vi "AndorSet.vi"(8 "error in":errorcluster, 9 "MultiTrack":cluster{"StartRow":i32, "EndRow":i32}={"StartRow"=1, "EndRow"=256}, 10 "AcqSet":T2={"openingtime"=20, "closingtime"=20, "ExposureTime"=0.01, "AccumCycTime"=0.0, "AccumCycNum"=1, "KineticNum"=1, "KineticTime"=0.0} {"KineticTime" format="%.2f"; "AccumCycTime" format="%.2f"; "ExposureTime" format="%.2f"}, 11 "Mode":T8={"AcqMode"=enum."Single Scan", "ReadMode"=enum."Image", "ShutterMode"=enum."Auto", "GateMode"=enum."TTL High", "TriggerMode"=enum."Internal"}) -> (0 "error out":errorcluster, 1 "SetStatus":bool, 2 "SetOut":T9, 3 "Timing":T1 {"kinetic" format="%.2f"; "accumulate" format="%.2f"; "exposure" format="%.2f"})   [LabVIEW 2014]
uses:
  <userlib>/atmcd64d.llb/AcquisitionMode_mode typedef.ctl
  <userlib>/atmcd64d.llb/ReadMode_mode typedef.ctl
  <userlib>/atmcd64d.llb/Shutter_mode typedef.ctl
  <userlib>/atmcd64d.llb/Shutter_type typedef.ctl
  <userlib>/atmcd64d.llb/TriggerMode_mode typedef.ctl
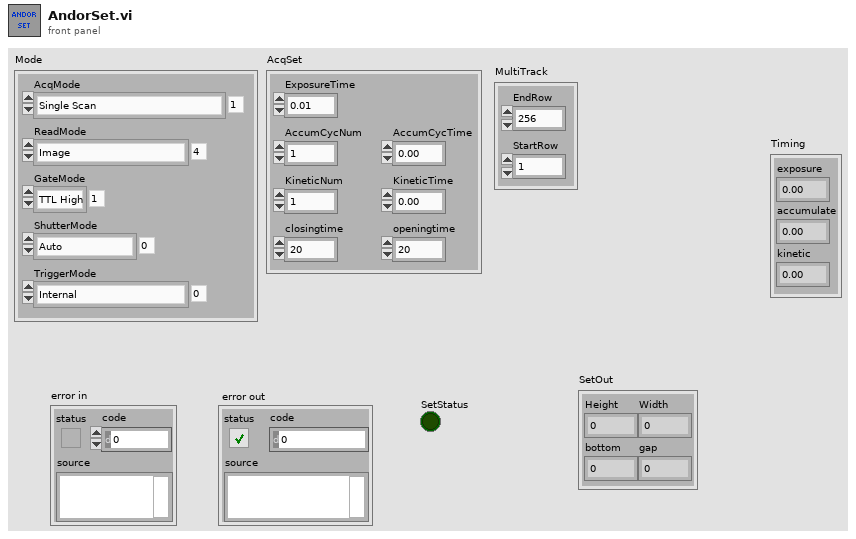
[diagram p1: front panel]
types:
  T1 = cluster{"exposure":sgl, "accumulate":sgl, "kinetic":sgl}
  T2 = cluster{"openingtime":i32, "closingtime":i32, "ExposureTime":sgl, "AccumCycTime":sgl, "AccumCycNum":i32, "KineticNum":i32, "KineticTime":sgl}
  T3 = typedef "AcquisitionMode_mode typedef.ctl" = enum16{"Reserved (0)", "Single Scan", "Accumulate", "Kinetics", "Fast Kinetics", "Run Till Abort", "Reserved (6)", "Reserved (7)", "Reserved (8)", "Time Delayed Integration"}
  T4 = typedef "ReadMode_mode typedef.ctl" = enum16{"Full Vertical Binning", "Multi-Track", "Random-Track", "Single-Track", "Image"}
  T5 = typedef "Shutter_mode typedef.ctl" = enum16{"Auto", "Open", "Close", "N/A (3)", "Open FVB Series", "Open Any Series"}
  T6 = typedef "Shutter_type typedef.ctl" = enum16{"TTL Low", "TTL High"}
  T7 = typedef "TriggerMode_mode typedef.ctl" = enum16{"Internal", "External", "N/A (2)", "N/A (3)", "N/A (4)", "N/A (5)", "External Start", "External Exposure (Bulb)", "N/A (8)", "External FVB EM", "Software", "N/A (11)", "External Charge Shifting"}
  T8 = cluster{"AcqMode":T3, "ReadMode":T4, "ShutterMode":T5, "GateMode":T6, "TriggerMode":T7}
  T9 = cluster{"Height":i32, "Width":i32, "bottom":i32, "gap":i32}
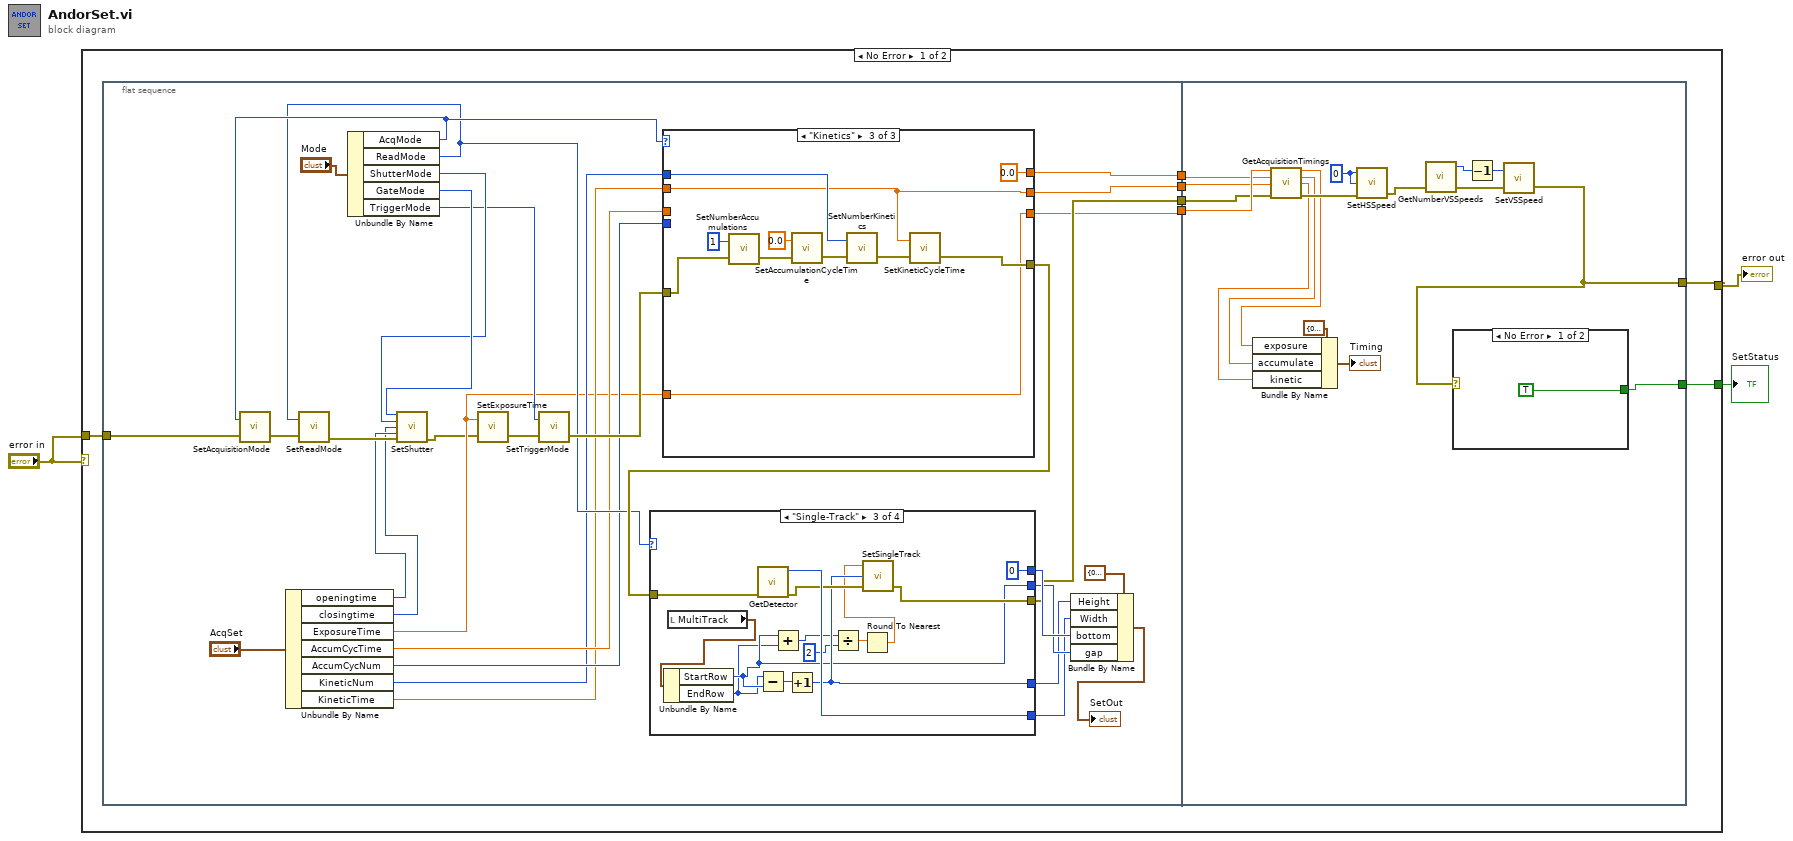
[diagram p0: block diagram]
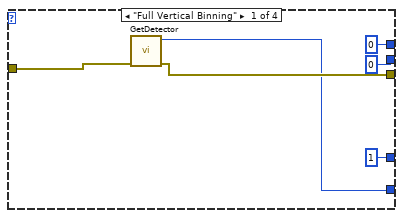
[diagram p2: hidden frame]
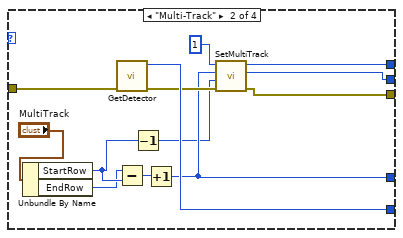
[diagram p3: hidden frame]
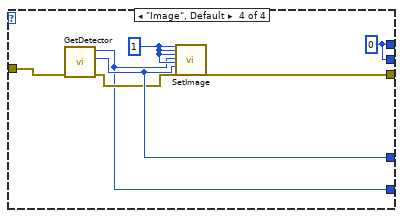
[diagram p4: hidden frame]
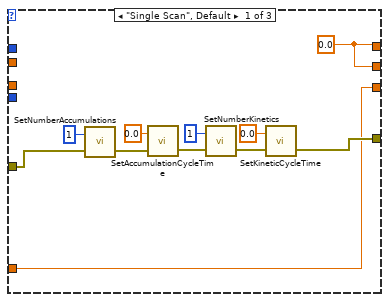
[diagram p5: hidden frame]
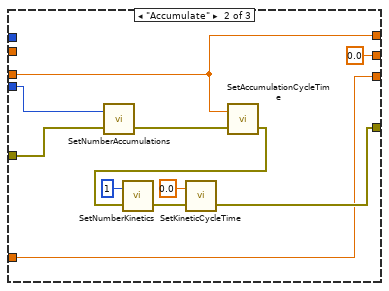
[diagram p6: hidden frame]
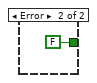
[diagram p7: hidden frame]
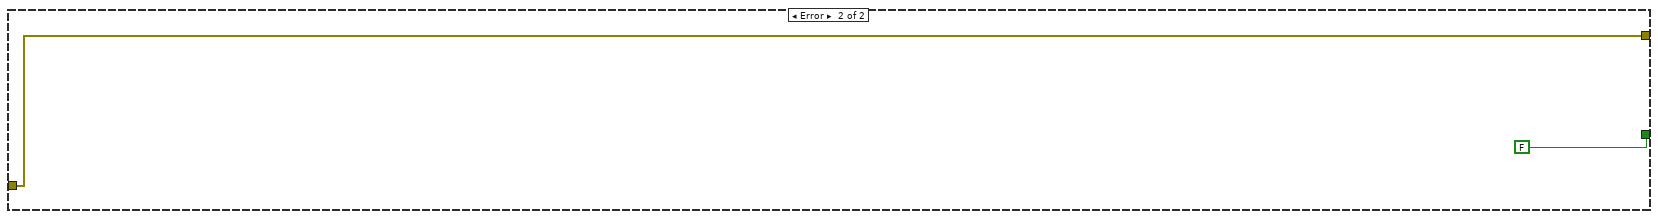
[diagram p8: hidden frame]
diagram:
  n1 = case shown="No Error" "error in" {
    tunnel: "error in" -> [w10 w134]
    tunnel: [w5 FALSE] -> w1
    tunnel: [w4 w134] -> w2
    frame No Error {
      n2 = flat-sequence {
        tunnel: w10 -> [w41]
        tunnel: [w30] -> w9
        tunnel: [w14] -> w8
        tunnel: [w13] -> w7
        tunnel: [w12] -> w6
        tunnel: w9 -> [w126]
        tunnel: w8 -> [w129]
        tunnel: w7 -> [w127]
        tunnel: w6 -> [w128]
        tunnel: [w124] -> w5
        tunnel: [w123] -> w4
        frame #0 {
          n3 = Unbundle By Name("AcqSet") -> ("openingtime"=w22:i32, "closingtime"=w21:i32, "ExposureTime"=w15:sgl, "AccumCycTime"=w19:sgl, "AccumCycNum"=w18:i32, "KineticNum"=w17:i32, "KineticTime"=w16:sgl)
          n4 = Unbundle By Name("Mode") -> ("AcqMode"=w26:T3, "ReadMode"=w25:T4, "ShutterMode"=w27:T5, "GateMode"=w28:T6, "TriggerMode"=w24:T7)
          n5 = call <userlib>:"SetAcquisitionMode.vi"("error in (no error)"=w41, "mode"=w26) -> ("error out"=w20:errorcluster)  [unwired: 1 out]
          n6 = call <userlib>:"SetReadMode.vi"("error in (no error)"=w20, "mode"=w25) -> ("error out"=w40:errorcluster)  [unwired: 1 out]
          n7 = call <userlib>:"SetShutter.vi"("type"=w28, "mode"=w27, "closingtime"=w21, "openingtime"=w22, "error in (no error)"=w40) -> ("error out"=w11:errorcluster)  [unwired: 9 in, 1 out]
          n8 = call <userlib>:"SetExposureTime.vi"("error in (no error)"=w11, "time"=w15) -> ("error out"=w39:errorcluster)  [unwired: 1 out]
          n9 = call <userlib>:"SetTriggerMode.vi"("error in (no error)"=w39, "mode"=w24) -> ("error out"=w38:errorcluster)  [unwired: 1 out]
          n10 = case shown="\"Kinetics\"" w26 {
            tunnel: w38 -> [w87 w103 w113]
            tunnel: [w86 w99 w108] -> w37
            tunnel: w19 -> [_ w95 _]
            tunnel: w18 -> [_ w96 _]
            tunnel: w17 -> [_ _ w107]
            tunnel: w16 -> [_ _ w106]
            tunnel: [w83 w95 sgl 0.0 ("AccumCycTime")] -> w13
            tunnel: [w83 sgl 0.0 ("exposure input") w106] -> w12
            tunnel: w15 -> [w82 w93 w105]
            tunnel: [w82 w93 w105] -> w14
            frame "Single Scan", Default {
              w83 = sgl 0.0 ("exposure input")
              n11 = call <userlib>:"SetNumberAccumulations.vi"("error in (no error)"=w87, "number"=1) -> ("error out"=w90:errorcluster)  [unwired: 1 out]
              n12 = call <userlib>:"SetAccumulationCycleTime.vi"("error in (no error)"=w90, "time"=sgl 0.0) -> ("error out"=w89:errorcluster)  [unwired: 1 out]
              n13 = call <userlib>:"SetNumberKinetics.vi"("error in (no error)"=w89, "number"=1) -> ("error out"=w92:errorcluster)  [unwired: 1 out]
              n14 = call <userlib>:"SetKineticCycleTime.vi"("error in (no error)"=w92, "time"=sgl 0.0) -> ("error out"=w86:errorcluster)  [unwired: 1 out]
            }
            frame "Accumulate" {
              n15 = call <userlib>:"SetNumberAccumulations.vi"("error in (no error)"=w103, "number"=w96) -> ("error out"=w102:errorcluster)  [unwired: 1 out]
              n16 = call <userlib>:"SetAccumulationCycleTime.vi"("error in (no error)"=w102, "time"=w95) -> ("error out"=w100:errorcluster)  [unwired: 1 out]
              n17 = call <userlib>:"SetNumberKinetics.vi"("error in (no error)"=w100, "number"=1) -> ("error out"=w101:errorcluster)  [unwired: 1 out]
              n18 = call <userlib>:"SetKineticCycleTime.vi"("error in (no error)"=w101, "time"=sgl 0.0) -> ("error out"=w99:errorcluster)  [unwired: 1 out]
            }
            frame "Kinetics" {
              n19 = call <userlib>:"SetNumberAccumulations.vi"("error in (no error)"=w113, "number"=1) -> ("error out"=w111:errorcluster)  [unwired: 1 out]
              n20 = call <userlib>:"SetAccumulationCycleTime.vi"("error in (no error)"=w111, "time"=sgl 0.0) -> ("error out"=w110:errorcluster)  [unwired: 1 out]
              n21 = call <userlib>:"SetNumberKinetics.vi"("error in (no error)"=w110, "number"=w107) -> ("error out"=w114:errorcluster)  [unwired: 1 out]
              n22 = call <userlib>:"SetKineticCycleTime.vi"("error in (no error)"=w114, "time"=w106) -> ("error out"=w108:errorcluster)  [unwired: 1 out]
            }
          }
          n23 = case shown="\"Single-Track\"" w25 {
            tunnel: w37 -> [w47 w60 w74 w81]
            tunnel: [1 ("ypixels") w55 w67 w79] -> w32
            tunnel: [w45 w59 w73 w76] -> w31
            tunnel: [w46 w51 w68 w77] -> w30
            tunnel: [0 ("bottom") w53 0 ("bottom") w75] -> w34
            tunnel: [0 ("bottom") w52 w66 w75] -> w33
            frame "Full Vertical Binning" {
              n24 = call <userlib>:"GetDetector.vi"("error in (no error)"=w47) -> ("error out"=w46:errorcluster, "xpixels"=w45:i32)  [unwired: 3 in, 2 out]
            }
            frame "Multi-Track" {
              n25 = Unbundle By Name("MultiTrack") -> ("StartRow"=w49:i32, "EndRow"=w48:i32)
              n26 = call <userlib>:"GetDetector.vi"("error in (no error)"=w60) -> ("error out"=w57:errorcluster, "xpixels"=w59:i32)  [unwired: 3 in, 2 out]
              n27 = Subtract(x=w48, y=w49) -> (x-y=w58:i32)
              n28 = Decrement(x=w49) -> (x-1=w54:i32)
              n29 = Increment(x=w58) -> (x+1=w55:i32)
              n30 = call <userlib>:"SetMultiTrack.vi"("error in (no error)"=w57, "offset"=w54, "height"=w55, "number"=1) -> ("error out"=w51:errorcluster, "gap"=w52:i32, "bottom"=w53:i32)  [unwired: 1 out]
            }
            frame "Single-Track" {
              n31 = local read "MultiTrack"() -> (w71:cluster{"StartRow":i32, "EndRow":i32})
              n32 = Unbundle By Name(w71) -> ("StartRow"=w66:i32, "EndRow"=w65:i32)
              n33 = call <userlib>:"GetDetector.vi"("error in (no error)"=w74) -> ("error out"=w69:errorcluster, "xpixels"=w73:i32)  [unwired: 3 in, 2 out]
              n34 = Subtract(x=w65, y=w66) -> (x-y=w72:i32)
              n35 = Add(x=w66, y=w65) -> (x+y=w64:i32)
              n36 = Increment(x=w72) -> (x+1=w67:i32)
              n37 = Divide(x=w64, y=2) -> (x/y=w62:dbl)
              n38 = Round To Nearest(number=w62) -> (nearest integer value=w61:dbl)
              n39 = call <userlib>:"SetSingleTrack.vi"("error in (no error)"=w69, "height"=w67, "centre"=w61) -> ("error out"=w68:errorcluster)  [unwired: 1 in, 1 out]
            }
            frame "Image", Default {
              w75 = 0 ("bottom")
              w80 = 1 ("hbin")
              n40 = call <userlib>:"GetDetector.vi"("error in (no error)"=w81) -> ("error out"=w78:errorcluster, "ypixels"=w79:i32, "xpixels"=w76:i32)  [unwired: 3 in, 1 out]
              n41 = call <userlib>:"SetImage.vi"("hbin"=w80, "vbin"=w80, "hstart"=w80, "hend"=w76, "vstart"=w80, "vend"=w79, "error in (no error)"=w78) -> ("error out"=w77:errorcluster)  [unwired: 19 in, 1 out]
            }
          }
          n42 = Bundle By Name(cluster=T9 {"Height"=0, "Width"=0, "bottom"=0, "gap"=0} ("SetOut"), "Height"=w32, "Width"=w31, "bottom"=w34, "gap"=w33) -> (→"SetOut":T9)
        }
        frame #1 {
          w130 = 0
          n43 = call <userlib>:"GetAcquisitionTimings.vi"("exposure input"=w129, "accumulate input"=w127, "kinetic input"=w128, "error in (no error)"=w126) -> ("exposure"=w117:sgl, "accumulate"=w116:sgl, "kinetic"=w115:sgl, "error out"=w125:errorcluster)  [unwired: 7 in, 1 out]
          n44 = Bundle By Name(cluster=T1 {"exposure"=0.0, "accumulate"=0.0, "kinetic"=0.0} ("Timing"), "exposure"=w117, "accumulate"=w116, "kinetic"=w115) -> (→"Timing":T1)
          n45 = call <userlib>:"SetHSSpeed.vi"("error in (no error)"=w125, "index"=w130, "type"=w130) -> ("error out"=w122:errorcluster)  [unwired: 1 in, 1 out]
          n46 = call <userlib>:"GetNumberVSSpeeds.vi"("error in (no error)"=w122) -> ("error out"=w121:errorcluster, "number"=w120:i32)  [unwired: 2 in, 1 out]
          n47 = Decrement(x=w120) -> (x-1=w131:i32)
          n48 = call <userlib>:"SetVSSpeed.vi"("error in (no error)"=w121, "index"=w131) -> ("error out"=w123:errorcluster)  [unwired: 1 out]
          n49 = case shown="No Error" w123 {
            tunnel: [TRUE FALSE] -> w124
            frame No Error {
            }
            frame Error {
            }
          }
        }
      }
    }
    frame Error {
    }
  }
  "error out" <- w2
  "SetStatus" <- w1
